vi "MH_BuildTimeTrace.vi"(6 "Trace2_In":u64[](array[numeric]), 7 "rawbits":u32[](array[numeric]), 8 "error in (no error)":errorcluster caption="entrée d'erreur (pas d'erreur)", 9 "Trace1_In":u64[](array[numeric]), 10 "Bin size(ps)":u64, 11 "oflcorr_in":u64) -> (0 "error out":errorcluster caption="sortie d'erreur", 1 "Trace1_Out":u64[](array[numeric]), 3 "oflcorr_out":u64, 4 "Trace2_Out":u64[](array[numeric]))   [LabVIEW 2019]
uses:
  84a42141-f272-44fd-88d0-bd2289331ced.vi
  68c86eef-f857-4804-b5e2-15e330fa4e9a.vi
panel:
  in  "TraceSize":u64
  out "LastIdx2":u64
  out "LastIdx1":u64
  in  "Trace2Ch":u32=2
  in  "Trace1Ch":u32=1
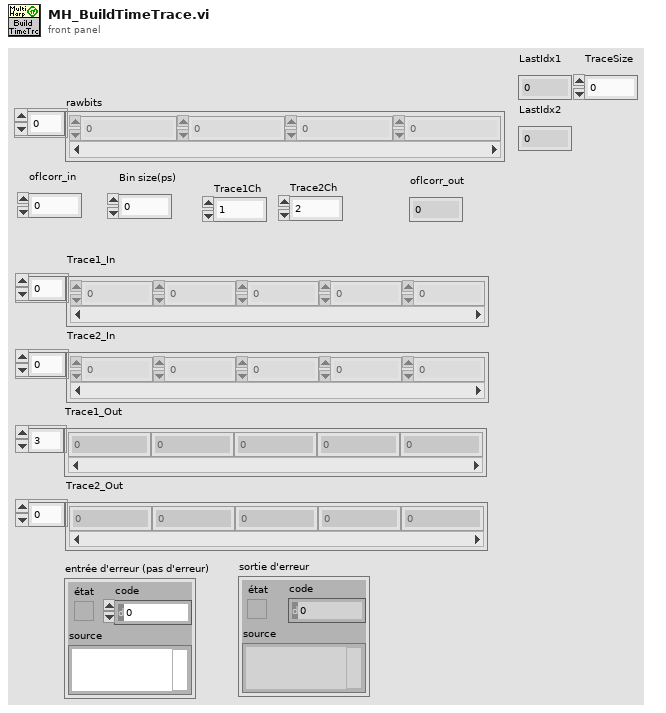
[diagram p1: front panel]
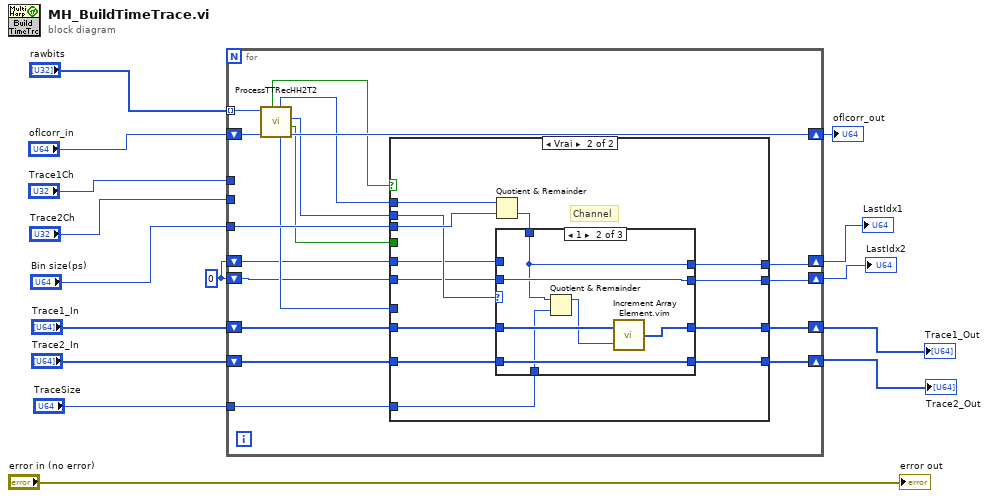
[diagram p0: block diagram]
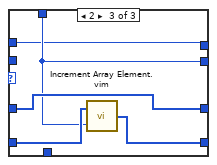
[diagram p4: hidden frame]
diagram:
  w4 = u64 0
  n1 = for {
    shift-right: [w33] -> w14
    shift-left: "oflcorr_in" -> [w32]
    tunnel: "rawbits" -> [w31] mode=indexing
    tunnel: "Trace1Ch" -> [_]
    tunnel: "Trace2Ch" -> [_]
    tunnel: "Bin size(ps)" -> [w29]
    shift-right: [w27] -> w8
    shift-left: "Trace1_In" -> [w28]
    shift-right: [w23] -> w6
    shift-left: "Trace2_In" -> [w24]
    shift-right: [w20] -> w2
    shift-left: w4 -> [w19]
    shift-right: [w18] -> w3
    shift-left: w4 -> [w17]
    tunnel: "TraceSize" -> [w16]
    n2 = call <userlib>:"ProcessTTRecHH2T2.vi"("oflcorr_in"=w32, "rawbits"=w31) -> ("oflcorr_out"=w33:u64, "is_marker"=w22:bool, "channel"=w25:u32, "markercode"=w21:u32, "truetime"=w30:u64, "is_photon"=w26:bool)  [unwired: 4 in]
    n3 = case shown="Vrai" w26 {
      tunnel: w30 -> [_ w50]
      tunnel: w29 -> [_ w49]
      tunnel: w28 -> [w37 w48]
      tunnel: [w37 w47] -> w27
      tunnel: w25 -> [_ w46]
      tunnel: w24 -> [w36 w45]
      tunnel: [w36 w44] -> w23
      tunnel: w22 -> [_ _]
      tunnel: w21 -> [_ _]
      tunnel: [w34 w42] -> w20
      tunnel: w19 -> [w34 w41]
      tunnel: [w35 w40] -> w18
      tunnel: w17 -> [w35 w39]
      tunnel: w16 -> [_ w38]
      frame False {
      }
      frame True {
        # "Channel"
        n4 = Quotient & Remainder(x=w50, y=w49) -> (floor(x/y)=w43:u64)  [unwired: 1 out]
        n5 = case shown="1" w46 {
          tunnel: w43 -> [_ w57 w63]
          tunnel: w48 -> [w54 w61 w66]
          tunnel: [w54 w60 w66] -> w47
          tunnel: w45 -> [w53 w59 w65]
          tunnel: [w53 w59 w64] -> w44
          tunnel: [w51 w58 w63] -> w42
          tunnel: w41 -> [w51 w58 _]
          tunnel: [w52 w57 w62] -> w40
          tunnel: w39 -> [w52 _ w62]
          tunnel: w38 -> [_ w56 _]
          frame 0, Default {
          }
          frame 1 {
            n6 = Quotient & Remainder(x=w57, y=w56) -> (x-y*floor(x/y)=w55:u64)  [unwired: 1 out]
            n7 = call "Increment Array Element.vim"("index"=w55, "array in"=w61) -> ("array out"=w60:u64[])
          }
          frame 2 {
            n8 = call "Increment Array Element.vim"("index"=w63, "array in"=w65) -> ("array out"=w64:u64[])
          }
        }
      }
    }
  }
  "oflcorr_out" <- w14
  "Trace1_Out" <- w8
  "Trace2_Out" <- w6
  "LastIdx1" <- w3
  "LastIdx2" <- w2
  "error out" <- "error in (no error)"
